vi "ColorGlobals.vi"() -> ()   [LabVIEW 2020]
panel:
  in  "Text":u32(colorbox)
  in  "Triple Quote":u32(colorbox)=9306312
  in  "Comment":u32(colorbox)=15665920
  in  "Python":u32(colorbox)=14453248
  in  "function":u32(colorbox)=239
  in  "Quote":u32(colorbox)=46086
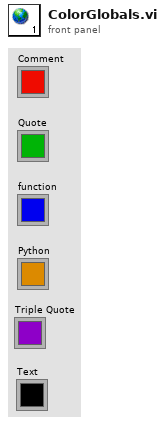
[diagram p1: front panel]
diagram:
